vi "DBLArrayToStr(cast).vi"(1 "DBL数组":dbl[](array[numeric])) -> (0 "字符串":string)   [LabVIEW 2012]
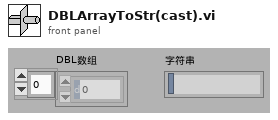
[diagram p1: front panel]
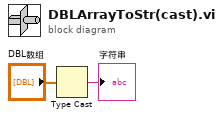
[diagram p0: block diagram]
diagram:
  n1 = Type Cast(x="DBL数组") -> (*(type *) &x=→"字符串":string)  [unwired: 1 in]
